vi "GetExpectedOutputs.vi"(11 "opinons":dbl[](array[numeric])) -> (1 "z":dbl[](array[numeric]), 2 "y":dbl[](array[numeric]), 3 "x":dbl[](array[numeric]))   [LabVIEW 2014]
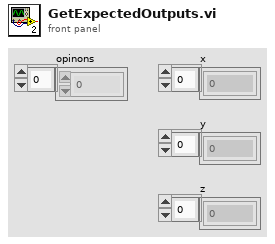
[diagram p1: front panel]
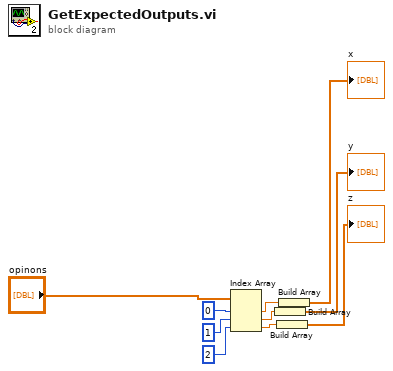
[diagram p0: block diagram]
diagram:
  n1 = Index Array(array="opinons", index #1=0 ("index"), index #2=1 ("index"), index #3=2 ("index")) -> (element #1=w5:dbl, element #2=w7:dbl, element #3=w6:dbl)
  n2 = Build Array(w7) -> (→"y":dbl[])
  n3 = Build Array(w6) -> (→"z":dbl[])
  n4 = Build Array(w5) -> (→"x":dbl[])
